vi "keithly one-time autorange.vi"(8 "error in":errorcluster, 11 "VISA in":refnum<visa-resource-name>="GPIB0::27::INSTR") -> (0 "error out":errorcluster, 2 "data":dbl[](array[numeric]), 3 "meter-VISA":refnum<visa-resource-name>)   [LabVIEW 2024]
doc: "VI intializes connection to Keithley 6517 picoampmeter (K6517) to read photodiode currents for reflectivity test station.\n\nK6517 must be connected to to PC via GPIB."
panel:
  # "Start Keithley 6517 Electrometer"
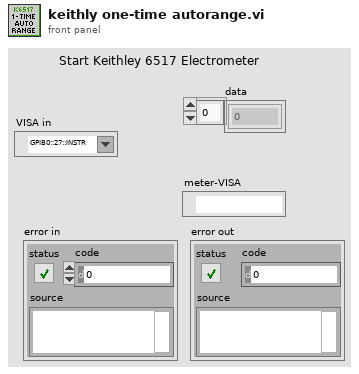
[diagram p1: front panel]
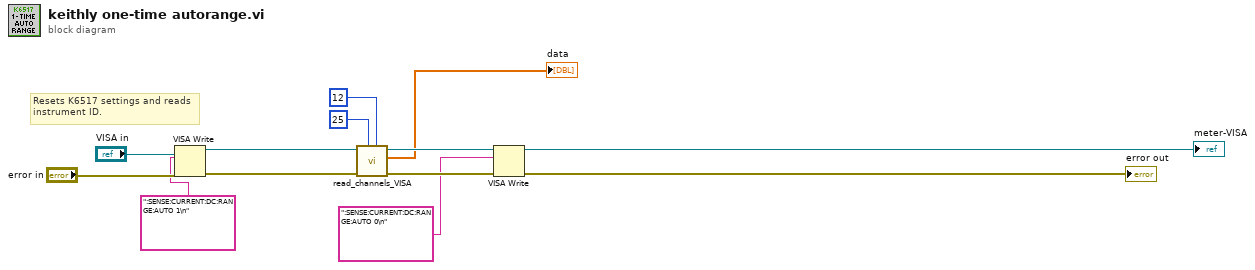
[diagram p0: block diagram]
diagram:
  # "Resets K6517 settings and reads\ninstrument ID."
  n1 = VISA Write(VISA resource name="VISA in", write buffer=":SENSE:CURRENT:DC:RANGE:AUTO 1\n", error in (no error)="error in") -> (VISA resource name out=w10:refnum<visa-resource-name>, error out=w6:errorcluster)  [unwired: 1 out]
  n2 = call "read_channels_VISA.vi"("postDAQ  wait ms"=u32 12, "preDAQ  wait ms"=u32 25, "VISA-in"=w10) -> ("data"=→"data":dbl[], "VISA-out"=w8:refnum<visa-resource-name>)  [unwired: 6 in, 1 out]
  n3 = VISA Write(VISA resource name=w8, write buffer=":SENSE:CURRENT:DC:RANGE:AUTO 0\n", error in (no error)=w6) -> (VISA resource name out=→"meter-VISA":refnum<visa-resource-name>, error out=→"error out":errorcluster)  [unwired: 1 out]
